vi "Camera.vi"(2 "Camera Queue":refnum<queue>, 3 "Wave Queue":refnum<queue>) -> (0 "error IO":errorcluster)   [LabVIEW 2016]
uses:
  controls/ModeEnum.ctl
  controls/Microscope Settings.ctl
  controls/ColourCalibration.ctl
  controls/CameraControlTypeDef.ctl
  controls/Stack_State.ctl
  controls/Stack Track.ctl
  <vilib>/vision/NI_Vision_Development_Module.lvlib
panel:
  out "Maximal Value":sgl
  in  "Display?":bool=TRUE
  out "Failed":bool
  out "Image":T1(plugin-control)
  out "FPS":dbl format="%#_3g"
  out "Image Path":path
  in  "Image Folder":path
  in  "Auto Contrast":bool
  out "Histogram":T2(graph)
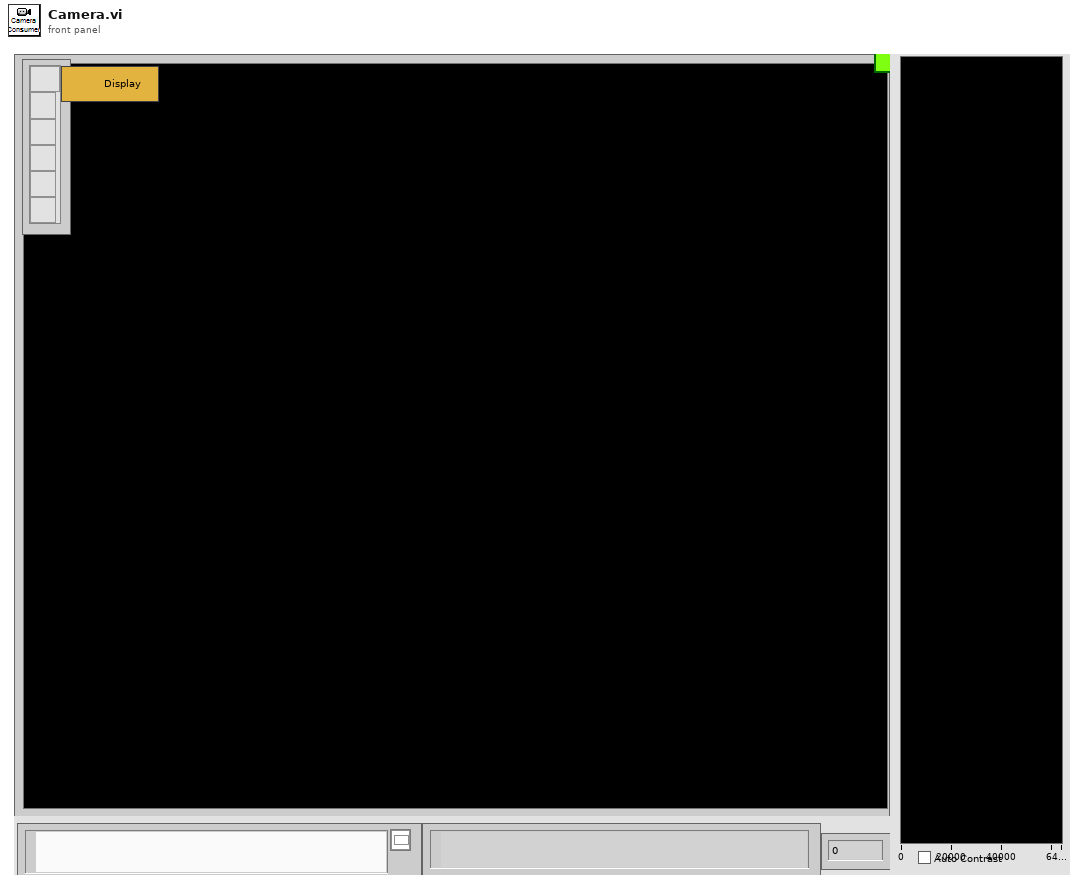
[diagram p1: front panel]
types:
  T1 = typedef "IMAQ Image.ctl" = refnum<image>
  T2 = cluster{"Starting Value":sgl, "Incremental Value":sgl, "Histogram":u32[]}
  T3 = typedef "Microscope Settings.ctl" = cluster{"Mode":enum16{"Brightfield", "X", "XY", "XYZ", "XYC", "XYCT", "XYZT", "XYZC", "Tweezers", "Virus"}, "Slit":cluster{"Scanning Mode":dbl, "Slit Width /%":dbl}, "Colour Channel":enum16{"1", "2", "3", "4", "5"}, "Colour":T4, "Exposure/ms":dbl, "Piezo Position /um":dbl, "ROI":cluster{"X":cluster{"Start /px":dbl, "Step /px":dbl, "Range /px":dbl}, "Y":cluster{"Start /px":dbl, "Step /px":dbl, "Range /px":dbl}, "Z ":cluster{"Start /um":dbl, "Step/um":dbl, "Range /um":dbl}, "T ":cluster{"Start /s":dbl, "Step /s":dbl, "Range /s":dbl}}, "Samples per millisecond":dbl, "Relax/ms":dbl, "Readout Direction":dbl, "Trigger Source":dbl, "Camera Delay /ms":dbl, "Under Scan /ms":dbl, "Slit Delay":dbl, "Waveforms":cluster{"Analogue Out":waveform(dbl)[], "Digital Out":digitalwaveform[]}}
  T4 = typedef "ColourCalibration.ctl" = cluster{"Colour":cluster{"Laser":enum16{"Brightfield", "445", "488", "561", "647"}, "Filter":u16}, "Calibration Coordinates":cluster{"Top Left":dbl[], "Top Right":dbl[], "Bottom Left":dbl[], "Bottom Right":dbl[]}, "Focus Offset /um":dbl}[]
  T5 = typedef "Image Type" = u32
  T6 = typedef "Stack_State.ctl" = cluster{"State":T7, "Image":u16[][], "Path":path}
  T7 = typedef "Stack Track.ctl" = enum16{"Idle", "STOP", "Display", "Save Image"}
  T8 = typedef "CameraControlTypeDef.ctl" = enum16{"Idle", "Init", "Close", "IntervalLineInt", "Ram Record", "HardDisk Record", "Disengage Update", "Update", "ROI", "Binning", "Scan Mode", "Trigger Mode", "Readout Mode", "Readout Direction", "Preview", "ROIWindow", "Trigger Source", "STOP"}
  T9 = cluster{"height":u32, "width":u32, "datatype":u32}
  T10 = typedef "ModeEnum.ctl" = enum16{"Idle", "Init", "generateWaves", "runWaves", "runWavesCont", "endWavesCont", "stop"}
  T11 = cluster{"Horizontal Offset":i32, "Vertical Offset":i32, "Horizontal Width":i32, "Vertical Width":i32}
  T12 = cluster{"Mode":u32, "Polarity":u32, "Times":u32, "Delay":dbl}
  T13 = cluster{"Start /px":dbl, "Step /px":dbl, "Range /px":dbl}
  T14 = cluster{"State":T7, "Data 16":u16[][], "Save to:":path}
  T15 = enum16{"Brightfield", "X", "XY", "XYZ", "XYC", "XYCT", "XYZT", "XYZC", "Tweezers", "Virus"}
  T16 = cluster{"histogram":u32[], "Minimal Value":sgl, "Maximal Value":sgl, "Starting Value":sgl, "Interval Width":sgl, "Mean Value":sgl, "Standard  Variation":sgl, "Area (pixels)":i32}
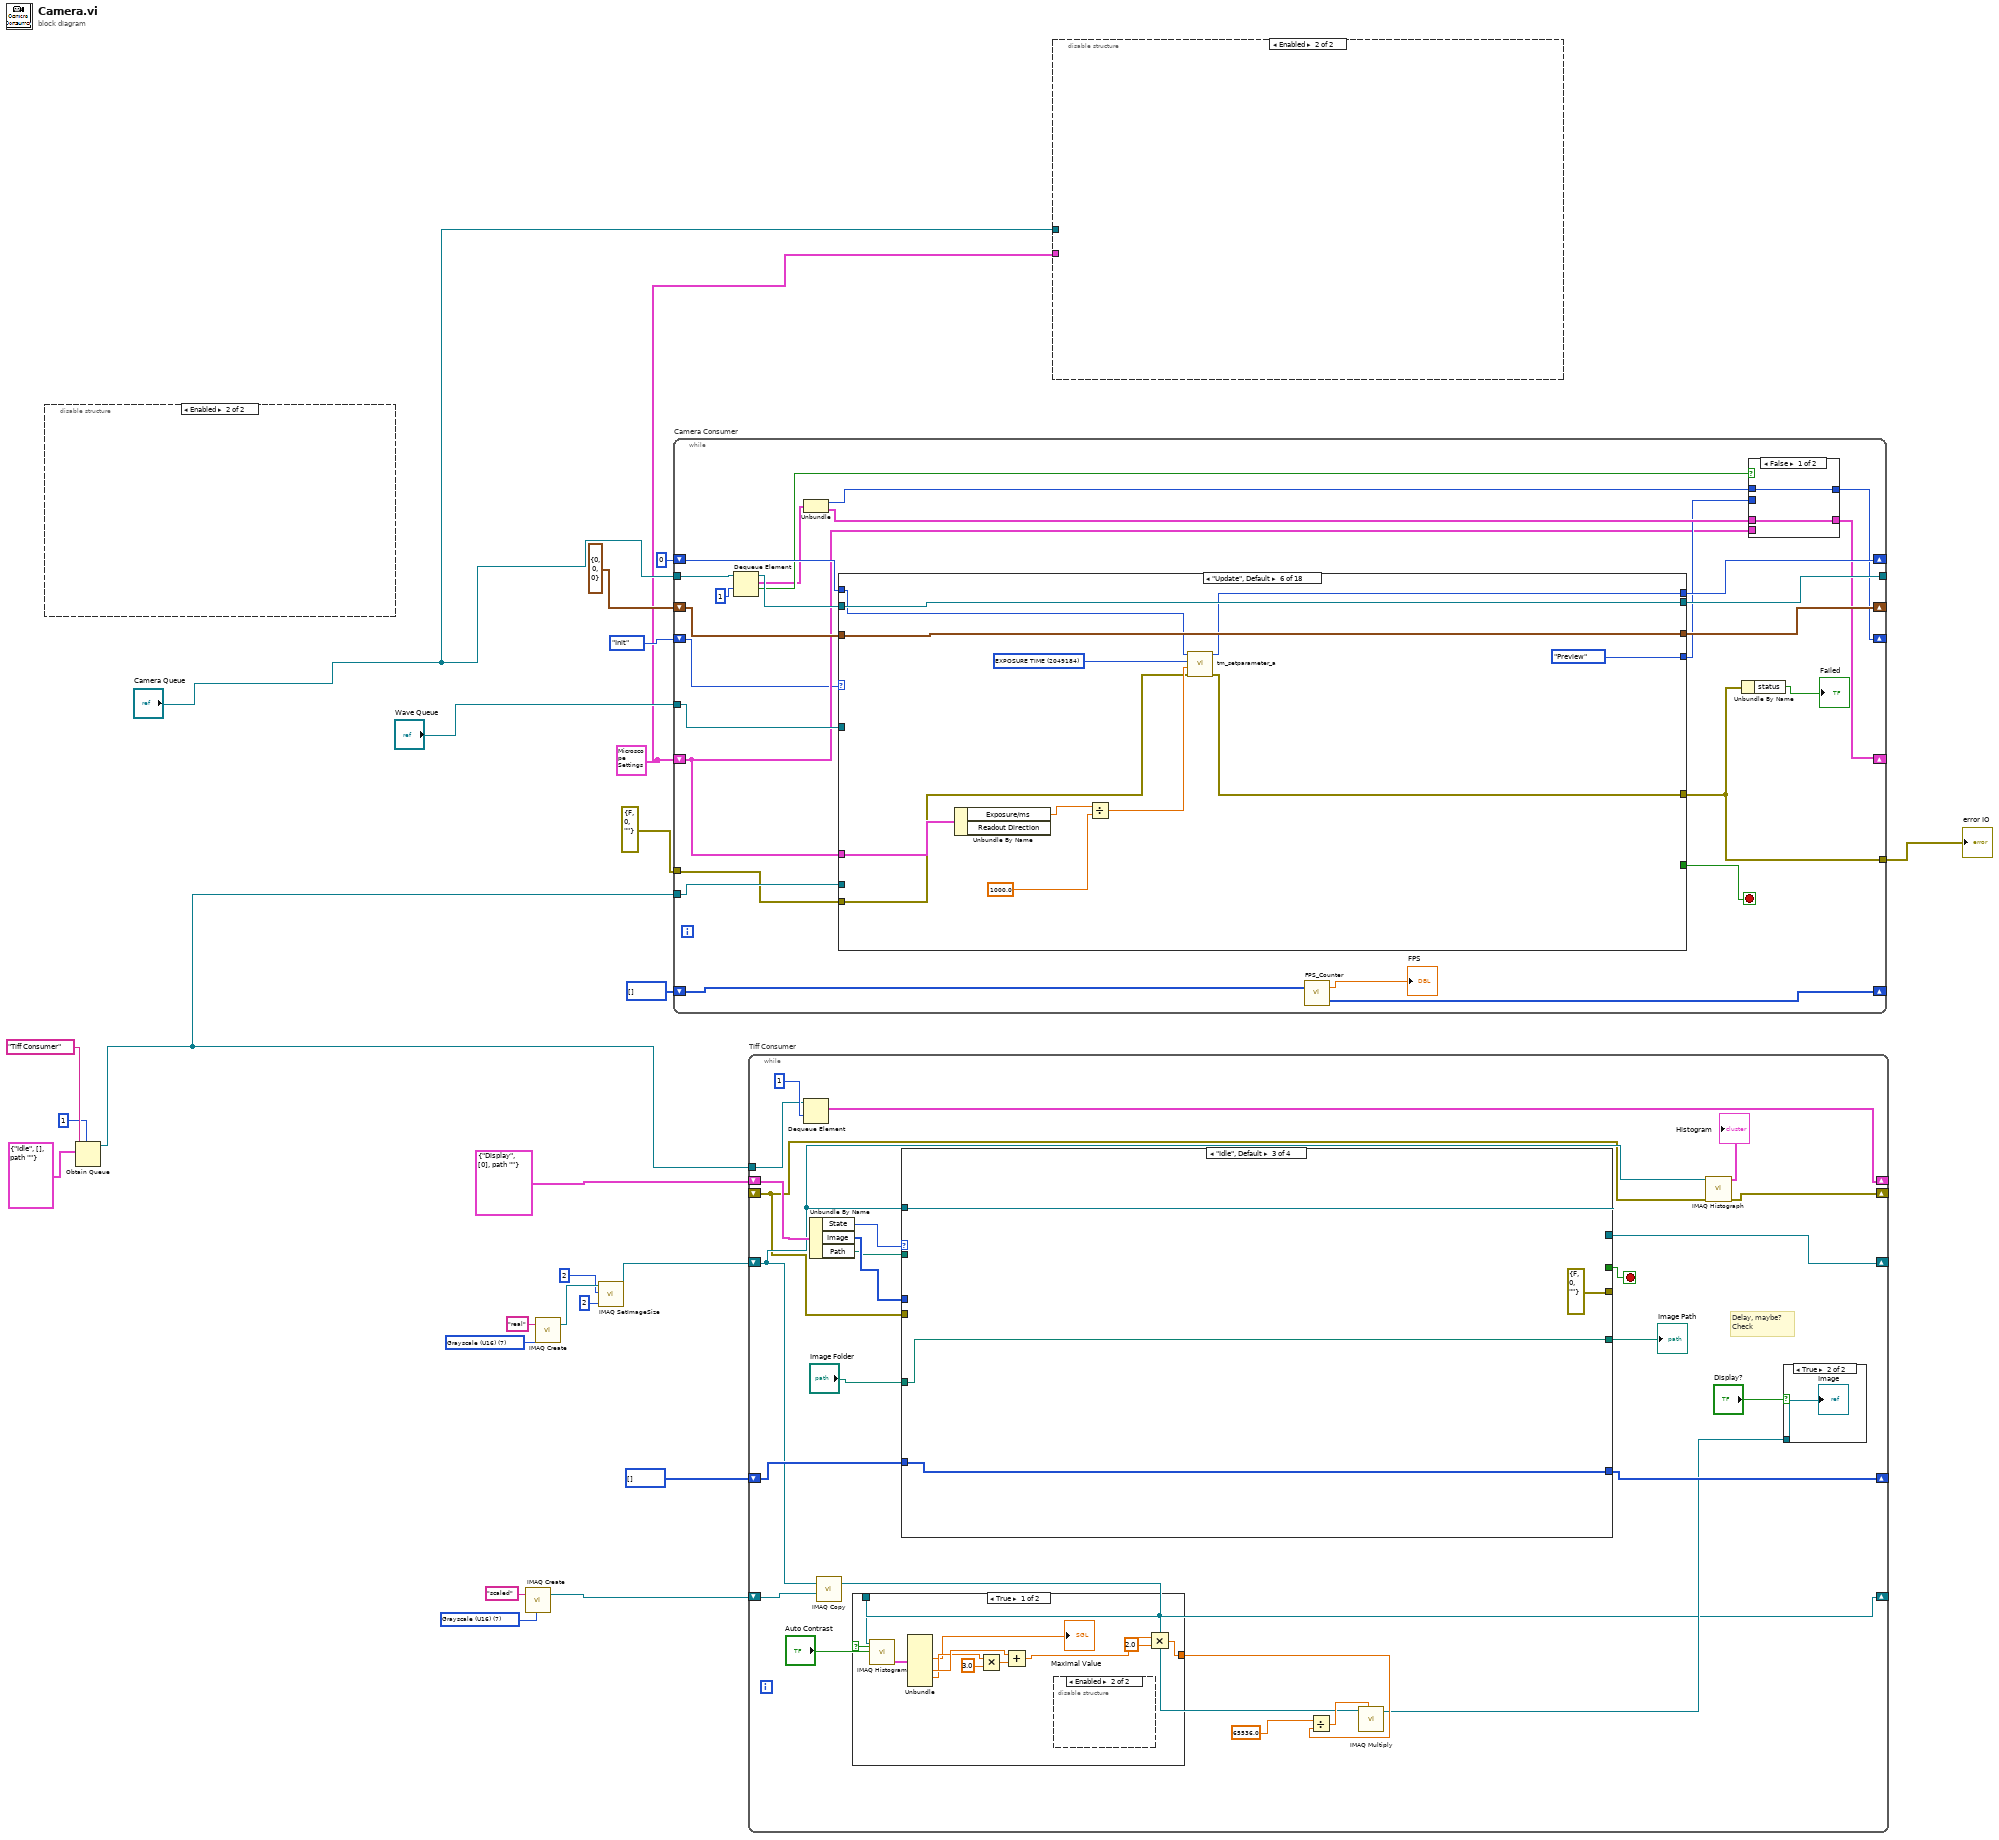
[diagram p0: block diagram]
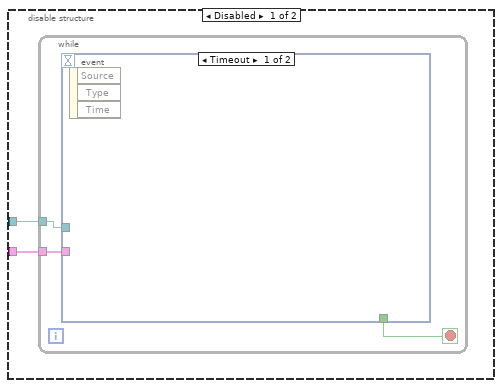
[diagram p2: hidden frame]
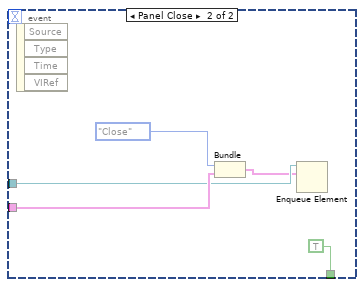
[diagram p3: hidden frame]
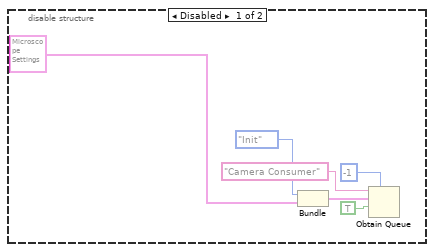
[diagram p4: hidden frame]
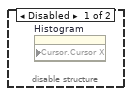
[diagram p5: hidden frame]
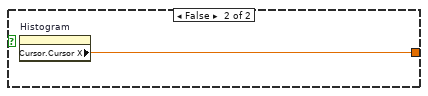
[diagram p6: hidden frame]
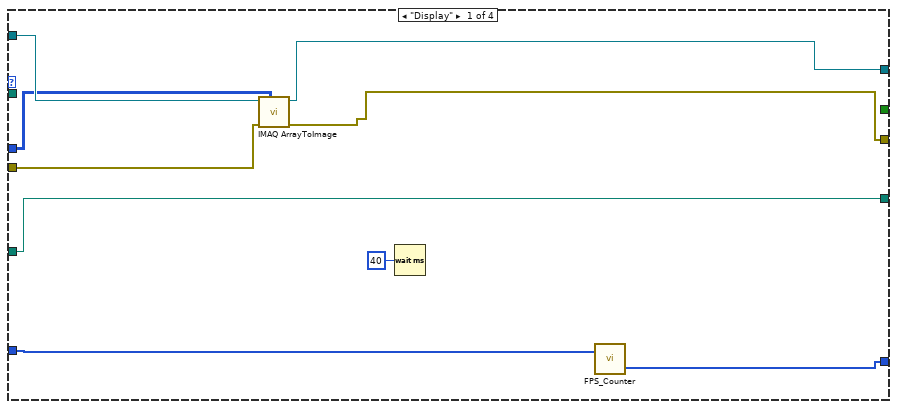
[diagram p8: hidden frame]
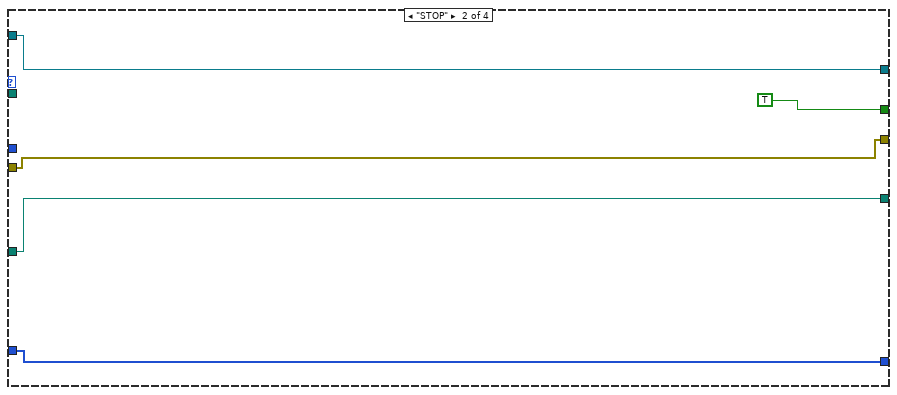
[diagram p9: hidden frame]
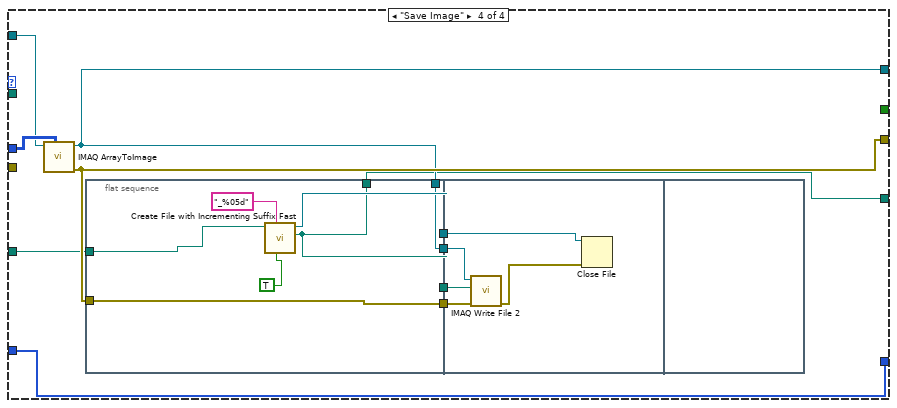
[diagram p10: hidden frame]
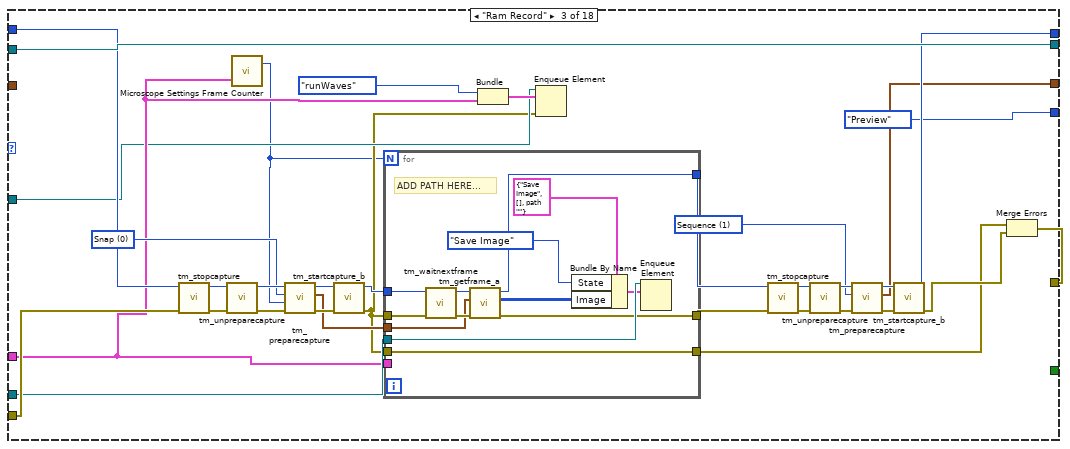
[diagram p13: hidden frame]
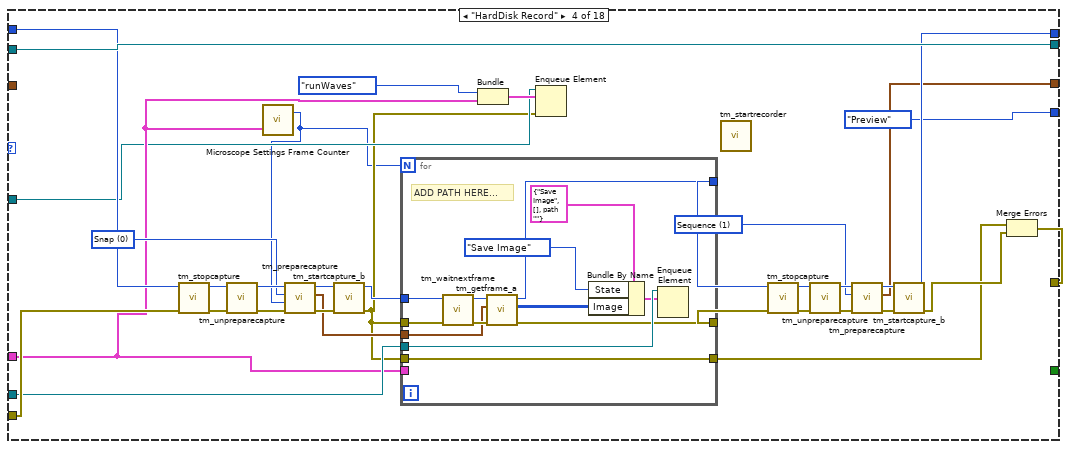
[diagram p14: hidden frame]
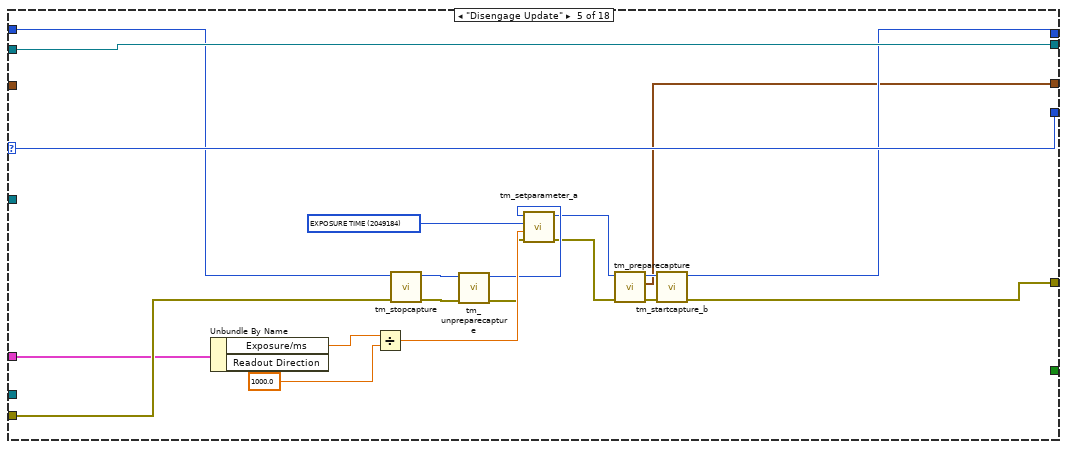
[diagram p15: hidden frame]
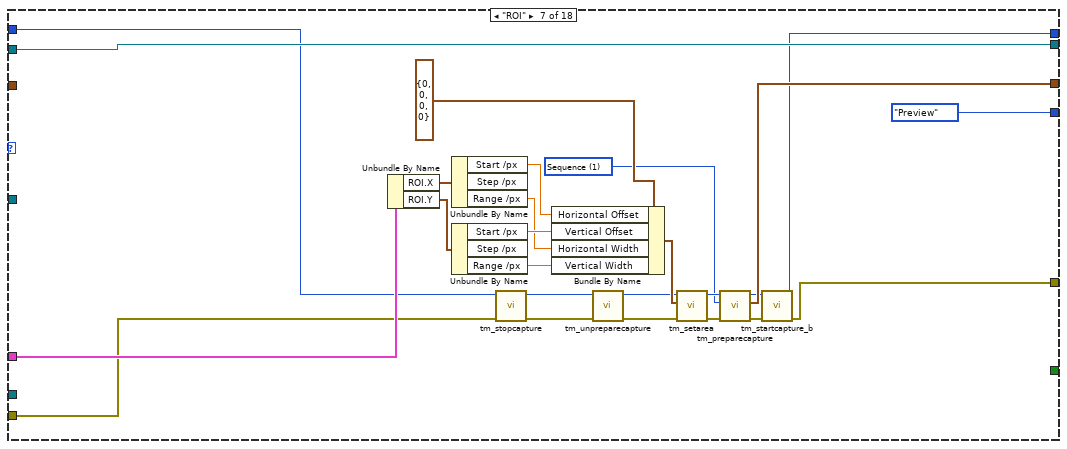
[diagram p16: hidden frame]
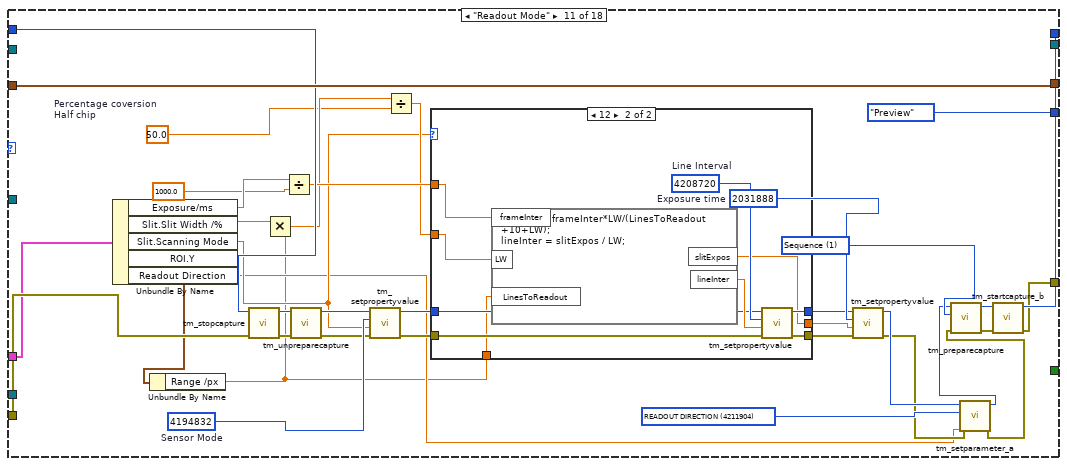
[diagram p20: hidden frame]
diagram:
  w1 = T3 {"Mode"=enum."X", "Slit"={"Scanning Mode"=12.0, "Slit Width /%"=5.0}, "Colour Channel"=enum."3", "Colour"=[], "Exposure/ms"=40.0, "Piezo Position /um"=10.0, "ROI"={"X"={"Start /px"=0.0, "Step /px"=1.0, "Range /px"=100.0}, "Y"={"Start /px"=0.0, "Step /px"=1.0, "Range /px"=100.0}, "Z "={"Start /um"=0.0, "Step/um"=1.0, "Range /um"=100.0}, "T "={"Start /s"=0.0, "Step /s"=1.0, "Range /s"=100.0}}, "Samples per millisecond"=100.0, "Relax/ms"=10000.0, "Readout Direction"=2.0, "Trigger Source"=2.0, "Camera Delay /ms"=11.0, "Under Scan /ms"=5.0, "Slit Delay"=100.0, "Waveforms"={"Analogue Out"=[{"t0"=timestamp(0 s since 1904-01-01), "dt"=1.0, "Y"=[]}, {"t0"=timestamp(0 s since 1904-01-01), "dt"=1.0, "Y"=[]}, {"t0"=timestamp(0 s since 1904-01-01), "dt"=1.0, "Y"=[]}], "Digital Out"=[{"t0"=timestamp(0 s since 1904-01-01), "dt"=0.0, "Y"={"transitions"=[], "data"=[]}}, {"t0"=timestamp(0 s since 1904-01-01), "dt"=0.0, "Y"={"transitions"=[], "data"=[]}}, {"t0"=timestamp(0 s since 1904-01-01), "dt"=0.0, "Y"={"transitions"=[], "data"=[]}}]}} ("Microscope Settings")
  w13 = T5 7 items=["Grayscale (U8)", "Grayscale (I16)", "Grayscale (SGL)", "Complex (CSG)", "RGB (U32)", "HSL (U32)", "RGB (U64)", "Grayscale (U16)"] ("Image Type")
  w24 = T5 7 items=["Grayscale (U8)", "Grayscale (I16)", "Grayscale (SGL)", "Complex (CSG)", "RGB (U32)", "HSL (U32)", "RGB (U64)", "Grayscale (U16)"] ("Image Type")
  n1 = disable-structure shown="Enabled" {
    frame Disabled {
      n2 = Bundle("Enum"=CameraControlTypeDef."Init", "Microscope Settings"=T3 {"Mode"=enum."X", "Slit"={"Scanning Mode"=12.0, "Slit Width /%"=5.0}, "Colour Channel"=enum."3", "Colour"=[{"Colour"={"Laser"=enum."561", "Filter"=4}, "Calibration Coordinates"={"Top Left"=[-4.418670520231216, -0.1592138728323702, 10.0], "Top Right"=[-9.501965317919073, -0.1592138728323702, 10.0], "Bottom Left"=[-4.4508670520231215, 0.0, 0.0], "Bottom Right"=[-9.53757225433526, 0.0, 0.0]}, "Focus Offset /um"=0.0}], "Exposure/ms"=40.0, "Piezo Position /um"=0.0, "ROI"={"X"={"Start /px"=0.0, "Step /px"=1.0, "Range /px"=2048.0}, "Y"={"Start /px"=0.0, "Step /px"=1.0, "Range /px"=2048.0}, "Z "={"Start /um"=0.0, "Step/um"=1.0, "Range /um"=100.0}, "T "={"Start /s"=0.0, "Step /s"=1.0, "Range /s"=100.0}}, "Samples per millisecond"=100.0, "Relax/ms"=10.0, "Readout Direction"=2.0, "Trigger Source"=2.0, "Camera Delay /ms"=11.0, "Under Scan /ms"=5.0, "Slit Delay"=100.0, "Waveforms"={"Analogue Out"=[{"t0"=timestamp(0 s since 1904-01-01), "dt"=1.0, "Y"=[]}, {"t0"=timestamp(0 s since 1904-01-01), "dt"=1.0, "Y"=[]}, {"t0"=timestamp(0 s since 1904-01-01), "dt"=1.0, "Y"=[]}], "Digital Out"=[{"t0"=timestamp(0 s since 1904-01-01), "dt"=0.0, "Y"={"transitions"=[], "data"=[]}}, {"t0"=timestamp(0 s since 1904-01-01), "dt"=0.0, "Y"={"transitions"=[], "data"=[]}}, {"t0"=timestamp(0 s since 1904-01-01), "dt"=0.0, "Y"={"transitions"=[], "data"=[]}}]}}) -> (w27:cluster{"Enum":T8, "Microscope Settings":T3})  [unwired: 1 in]
      n3 = Obtain Queue(max queue size (-1, unlimited)=-1, name (unnamed)="Camera Consumer", element data type=w27, create if not found? (T)=TRUE) -> ()  [unwired: 1 in, 3 out]
    }
    frame Enabled {
    }
  }
  n4 = Obtain Queue(max queue size (-1, unlimited)=1, name (unnamed)="Tiff Consumer", element data type=T6 {"State"=enum."Idle", "Image"=[], "Path"=path ""} ("input cluster")) -> (queue out=w14:refnum<queue>)  [unwired: 2 in, 2 out]
  n5 = call "IMAQ Create"("Image Name"="scaled", "Image Type"=w13) -> ("New Image"=w11:T1)  [unwired: 3 in, 1 out]
  n6 = call "IMAQ Create"("Image Name"="real", "Image Type"=w24) -> ("New Image"=w7:T1)  [unwired: 3 in, 1 out]
  n7 = call "IMAQ SetImageSize"("Y Resolution"=2, "X Resolution"=2, "Image"=w7) -> ("Image Out"=w6:T1)  [unwired: 2 in, 1 out]
  n8 = while "Camera Consumer" {
    tunnel: errorcluster {"status"=FALSE, "code"=0, "source"=""} ("error IO") -> [w42]
    tunnel: [w44] -> w17
    tunnel: "Camera Queue" -> [w50]
    tunnel: [w56] -> _
    shift-right: [w36] -> _
    shift-left: CameraControlTypeDef."Init" ("Enum") -> [w34]
    tunnel: w14 -> [w48]
    shift-right: [w54] -> _
    shift-left: u32 0 ("Handle out") -> [w55]
    tunnel: "Wave Queue" -> [w47]
    shift-right: [w53] -> _
    shift-left: T9 {"height"=0, "width"=0, "datatype"=0} ("Buffer Info") -> [w52]
    shift-right: [w37] -> _
    shift-left: w1 -> [w35]
    shift-right: [w32] -> _
    shift-left: u32[] [] ("Array out") -> [w33]
    stop <- w45 stop-if-true
    n9 = Dequeue Element(queue=w50, timeout in ms (-1)=1) -> (queue out=w49:refnum<queue>, element=w41:cluster{"Enum":T8, "Microscope Settings":T3}, timed out?=w46:bool)  [unwired: 1 in, 1 out]
    n10 = Unbundle(w41) -> ("Enum"=w40:T8, "Microscope Settings"=w39:T3)
    n11 = case shown="\"Update\", Default" w34 {
      selector: w34 -> [w60 w65 _ _ w179 _ _ w221 w226 w231 _ w287 _ w318 _ _ _ _]
      tunnel: w49 -> [w59 w66 w100 w147 w180 w192 w217 w222 w227 w232 _ w283 w299 w320 w331 w385 w405 w442]
      tunnel: [w59 w66 w100 w147 w180 w192 w217 w222 w227 w232 _ w283 w299 w320 w330 _ _ w442] -> w56
      tunnel: w42 -> [w61 w64 w99 w146 w171 w182 w195 w220 w225 w230 w265 w286 w292 w317 w321 w390 w410 w433]
      tunnel: [w61 w64 w77 w124 w170 w181 w198 w220 w225 w230 w242 w286 w291 w317 w334 w384 w404 w434] -> w44
      tunnel: [w60 w65 CameraControlTypeDef."Preview" ("Enum") CameraControlTypeDef."Preview" ("Enum") w179 CameraControlTypeDef."Preview" ("Enum") CameraControlTypeDef."Preview" ("Enum") w221 w226 w231 CameraControlTypeDef."Preview" ("Enum") w287 CameraControlTypeDef."Preview" ("Enum") w318 CameraControlTypeDef."Trigger Source" ("Enum") CameraControlTypeDef."Idle" ("Enum") CameraControlTypeDef."Idle" ("Enum") w424] -> w38
      tunnel: w55 -> [w58 w63 w83 w130 w174 w190 w197 w219 w224 w229 w267 w285 w298 w319 _ w381 w401 w436]
      tunnel: [w58 w63 w82 w129 w173 w189 w200 w219 w224 w229 w243 w285 w296 w319 w336 w381 w401 w435] -> w54
      tunnel: [w57 w62 w79 w126 w172 w191 w202 w218 w223 w228 w269 w284 w294 w316 w333 w382 w402 w437] -> w53
      tunnel: w52 -> [w57 w62 _ _ _ w191 _ w218 w223 w228 w269 w284 w294 w316 _ w382 w402 _]
      tunnel: w48 -> [_ _ w92 w139 _ _ _ _ _ _ _ _ w293 _ _ w375 w399 _]
      tunnel: w35 -> [_ _ w70 w117 w167 w188 w216 _ _ _ w264 _ _ _ w332 _ _ w426]
      tunnel: w47 -> [_ _ w69 w116 _ _ _ _ _ _ _ _ _ _ _ _ _ _]
      tunnel: [_ _ _ _ _ _ _ _ _ _ _ _ _ _ _ TRUE FALSE _] -> w45
      frame "Idle" {
      }
      frame "IntervalLineInt" {
      }
      frame "Ram Record" {
        w96 = 0 items=["Snap", "Sequence"] ("Capture mode")
        w80 = 1 items=["Snap", "Sequence"] ("Capture mode")
        n12 = call <userlib>:"tm_stopcapture.vi"("error in (no error)"=w99, "Handle in"=w83) -> ("error out"=w75:errorcluster, "Handle out"=w76:u32)  [unwired: 8 in]
        n13 = call <userlib>:"tm_unpreparecapture.vi"("error in (no error)"=w75, "Handle in"=w76) -> ("error out"=w98:errorcluster, "Handle out"=w97:u32)  [unwired: 8 in]
        n14 = call "Microscope Settings Frame Counter.vi"("Microscope Settings in"=w70) -> ("Camera Prepare"=w67:i32)  [unwired: 1 in, 1 out]
        n15 = call <userlib>:"tm_preparecapture.vi"("error in (no error)"=w98, "Frames"=w67, "Capture mode"=w96, "Handle in"=w97) -> ("error out"=w94:errorcluster, "Buffer Info"=w81:T9, "Handle out"=w95:u32)  [unwired: 4 in, 1 out]
        n16 = call <userlib>:"tm_startcapture_b.vi"("error in (no error)"=w94, "Handle in"=w95) -> ("error out"=w68:errorcluster, "Handle out"=w93:u32)  [unwired: 8 in]
        n17 = for {
          N: w67 -> [_]
          tunnel: w68 -> [w113]
          tunnel: w93 -> [w112]
          tunnel: w92 -> [w108]
          tunnel: [w106] -> w88
          tunnel: [w105] -> w87
          tunnel: w81 -> [w104]
          tunnel: w68 -> [w101]
          tunnel: w70 -> [_]
          tunnel: [w101] -> w74
          # "ADD PATH HERE..."
          n18 = call <userlib>:"tm_waitnextframe.vi"("error in (no error)"=w113, "Handle in"=w112) -> ("error out"=w111:errorcluster, "Handle out"=w110:u32)  [unwired: 6 in, 2 out]
          n19 = call <userlib>:"tm_getframe_a.vi"("error in (no error)"=w111, "Buffer Info"=w104, "Handle in"=w110) -> ("error out"=w106:errorcluster, "Data 16"=w103:u16[][], "Handle out"=w105:u32)  [unwired: 4 in, 2 out]
          n20 = Bundle By Name(cluster=T6 {"State"=enum."Save Image", "Image"=[], "Path"=path ""} ("element"), "State"=Stack_Track."Save Image", "Image"=w103) -> (w107:T6)
          n21 = Enqueue Element(queue=w108, element=w107) -> ()  [unwired: 2 in, 3 out]
        }
        n22 = Bundle("Mode"=ModeEnum."runWaves", "Microscope Settings"=w70) -> (w72:cluster{"Mode":T10, "Microscope Settings":T3})  [unwired: 1 in]
        n23 = Enqueue Element(queue=w69, element=w72, error in (no error)=w68) -> ()  [unwired: 1 in, 3 out]
        n24 = call <userlib>:"tm_stopcapture.vi"("error in (no error)"=w88, "Handle in"=w87) -> ("error out"=w89:errorcluster, "Handle out"=w86:u32)  [unwired: 8 in]
        n25 = call <userlib>:"tm_unpreparecapture.vi"("error in (no error)"=w89, "Handle in"=w86) -> ("error out"=w90:errorcluster, "Handle out"=w85:u32)  [unwired: 8 in]
        n26 = call <userlib>:"tm_preparecapture.vi"("error in (no error)"=w90, "Capture mode"=w80, "Handle in"=w85) -> ("error out"=w91:errorcluster, "Buffer Info"=w79:T9, "Handle out"=w84:u32)  [unwired: 5 in, 1 out]
        n27 = call <userlib>:"tm_startcapture_b.vi"("error in (no error)"=w91, "Handle in"=w84) -> ("error out"=w78:errorcluster, "Handle out"=w82:u32)  [unwired: 8 in]
        n28 = Merge Errors(w74, w78) -> (w77:errorcluster)
      }
      frame "HardDisk Record" {
        w143 = 0 items=["Snap", "Sequence"] ("Capture mode")
        w127 = 1 items=["Snap", "Sequence"] ("Capture mode")
        n29 = call <userlib>:"tm_stopcapture.vi"("error in (no error)"=w146, "Handle in"=w130) -> ("error out"=w122:errorcluster, "Handle out"=w123:u32)  [unwired: 8 in]
        n30 = call <userlib>:"tm_unpreparecapture.vi"("error in (no error)"=w122, "Handle in"=w123) -> ("error out"=w145:errorcluster, "Handle out"=w144:u32)  [unwired: 8 in]
        n31 = call "Microscope Settings Frame Counter.vi"("Microscope Settings in"=w117) -> ("Camera Prepare"=w114:i32)  [unwired: 1 in, 1 out]
        n32 = call <userlib>:"tm_preparecapture.vi"("error in (no error)"=w145, "Frames"=w114, "Capture mode"=w143, "Handle in"=w144) -> ("error out"=w141:errorcluster, "Buffer Info"=w128:T9, "Handle out"=w142:u32)  [unwired: 4 in, 1 out]
        n33 = call <userlib>:"tm_startcapture_b.vi"("error in (no error)"=w141, "Handle in"=w142) -> ("error out"=w115:errorcluster, "Handle out"=w140:u32)  [unwired: 8 in]
        n34 = for {
          N: w114 -> [_]
          tunnel: w115 -> [w160]
          tunnel: w140 -> [w159]
          tunnel: w139 -> [w155]
          tunnel: [w153] -> w135
          tunnel: [w152] -> w134
          tunnel: w128 -> [w151]
          tunnel: w115 -> [w148]
          tunnel: w117 -> [_]
          tunnel: [w148] -> w121
          # "ADD PATH HERE..."
          n35 = call <userlib>:"tm_waitnextframe.vi"("error in (no error)"=w160, "Handle in"=w159) -> ("error out"=w158:errorcluster, "Handle out"=w157:u32)  [unwired: 6 in, 2 out]
          n36 = call <userlib>:"tm_getframe_a.vi"("error in (no error)"=w158, "Buffer Info"=w151, "Handle in"=w157) -> ("error out"=w153:errorcluster, "Data 16"=w150:u16[][], "Handle out"=w152:u32)  [unwired: 4 in, 2 out]
          n37 = Bundle By Name(cluster=T6 {"State"=enum."Save Image", "Image"=[], "Path"=path ""} ("element"), "State"=Stack_Track."Save Image", "Image"=w150) -> (w154:T6)
          n38 = Enqueue Element(queue=w155, element=w154) -> ()  [unwired: 2 in, 3 out]
        }
        n39 = Bundle("Mode"=ModeEnum."runWaves", "Microscope Settings"=w117) -> (w119:cluster{"Mode":T10, "Microscope Settings":T3})  [unwired: 1 in]
        n40 = Enqueue Element(queue=w116, element=w119, error in (no error)=w115) -> ()  [unwired: 1 in, 3 out]
        n41 = call <userlib>:"tm_startrecorder.vi"() -> ()  [unwired: 10 in, 2 out]
        n42 = call <userlib>:"tm_stopcapture.vi"("error in (no error)"=w135, "Handle in"=w134) -> ("error out"=w136:errorcluster, "Handle out"=w133:u32)  [unwired: 8 in]
        n43 = call <userlib>:"tm_unpreparecapture.vi"("error in (no error)"=w136, "Handle in"=w133) -> ("error out"=w137:errorcluster, "Handle out"=w132:u32)  [unwired: 8 in]
        n44 = call <userlib>:"tm_preparecapture.vi"("error in (no error)"=w137, "Capture mode"=w127, "Handle in"=w132) -> ("error out"=w138:errorcluster, "Buffer Info"=w126:T9, "Handle out"=w131:u32)  [unwired: 5 in, 1 out]
        n45 = call <userlib>:"tm_startcapture_b.vi"("error in (no error)"=w138, "Handle in"=w131) -> ("error out"=w125:errorcluster, "Handle out"=w129:u32)  [unwired: 8 in]
        n46 = Merge Errors(w121, w125) -> (w124:errorcluster)
      }
      frame "Disengage Update" {
        w169 = u32 2049184 items=["SENSOR MODE"=4212128, "CCD MODE"=4212384, "READOUT MODE"=4211872, "ACTIVE VIEW INDEX"=4343136, "BITS PER CHANNEL"=4342976, "IMAGE PIXEL TYPE"=4343296, "BINNING"=4215968, "EXPOSURE TIME"=2049184, "CONTRAST GAIN"=3163312, "CONTRAST OFFSET"=3163328, "LIGHT MODE"=2114720, "SENSITIVITY"=2114992, "PHOTON IMAGING MODE"=2115200, "HIGH DYNAMIC RANGE MODE"=3163360, "WHITE BALANCE"=3163568, "TEMPERATURE"=2115232, "TEMPERATURE TARGET"=2115264, "SENSOR COOLER FAN"=2115296, "LINEBUNDLE HEIGHT"=4212192, "MECHANICAL SHUTTER"=2115488, "BACK FOCUS POSITION"=8422304, "TRIGGER CONNECTOR"=1066432, "TRIGGER SOURCE"=1066144, "OUTPUT TRIGGER SOURCE"=1852576, "TRIGGER GLOBAL EXPOSURE"=2049680, "FIRST TRIGGER BEHAVIOR"=2049696, "CHANNEL SYNC"=1852352, "READOUT DIRECTION"=4211904, "PRE HSYNC COUNT"=1852704, "INTERNAL LINE SPEED"=4226000, "INTERNAL LINE INTERVAL"=4226016] ("Parameter")
        n47 = Unbundle By Name(w167) -> ("Exposure/ms"=w166:dbl)  [unwired: 1 out]
        n48 = Divide(x=w166, y=1000.0) -> (x/y=w165:dbl)
        n49 = call <userlib>:"tm_stopcapture.vi"("error in (no error)"=w171, "Handle in"=w174) -> ("error out"=w177:errorcluster, "Handle out"=w176:u32)  [unwired: 8 in]
        n50 = call <userlib>:"tm_unpreparecapture.vi"("error in (no error)"=w177, "Handle in"=w176) -> ("error out"=w161:errorcluster, "Handle out"=w164:u32)  [unwired: 8 in]
        n51 = call <userlib>:"tm_setparameter_a.vi"("error in (no error)"=w161, "Value in"=w165, "Parameter"=w169, "Handle in"=w164) -> ("error out"=w162:errorcluster, "Handle out"=w163:u32)  [unwired: 6 in]
        n52 = call <userlib>:"tm_preparecapture.vi"("error in (no error)"=w162, "Handle in"=w163) -> ("error out"=w178:errorcluster, "Buffer Info"=w172:T9, "Handle out"=w175:u32)  [unwired: 6 in, 1 out]
        n53 = call <userlib>:"tm_startcapture_b.vi"("error in (no error)"=w178, "Handle in"=w175) -> ("error out"=w170:errorcluster, "Handle out"=w173:u32)  [unwired: 8 in]
      }
      frame "Update", Default {
        w185 = u32 2049184 items=["SENSOR MODE"=4212128, "CCD MODE"=4212384, "READOUT MODE"=4211872, "ACTIVE VIEW INDEX"=4343136, "BITS PER CHANNEL"=4342976, "IMAGE PIXEL TYPE"=4343296, "BINNING"=4215968, "EXPOSURE TIME"=2049184, "CONTRAST GAIN"=3163312, "CONTRAST OFFSET"=3163328, "LIGHT MODE"=2114720, "SENSITIVITY"=2114992, "PHOTON IMAGING MODE"=2115200, "HIGH DYNAMIC RANGE MODE"=3163360, "WHITE BALANCE"=3163568, "TEMPERATURE"=2115232, "TEMPERATURE TARGET"=2115264, "SENSOR COOLER FAN"=2115296, "LINEBUNDLE HEIGHT"=4212192, "MECHANICAL SHUTTER"=2115488, "BACK FOCUS POSITION"=8422304, "TRIGGER CONNECTOR"=1066432, "TRIGGER SOURCE"=1066144, "OUTPUT TRIGGER SOURCE"=1852576, "TRIGGER GLOBAL EXPOSURE"=2049680, "FIRST TRIGGER BEHAVIOR"=2049696, "CHANNEL SYNC"=1852352, "READOUT DIRECTION"=4211904, "PRE HSYNC COUNT"=1852704, "INTERNAL LINE SPEED"=4226000, "INTERNAL LINE INTERVAL"=4226016] ("Parameter")
        n54 = Unbundle By Name(w188) -> ("Exposure/ms"=w187:dbl)  [unwired: 1 out]
        n55 = Divide(x=w187, y=1000.0) -> (x/y=w184:dbl)
        n56 = call <userlib>:"tm_setparameter_a.vi"("error in (no error)"=w182, "Value in"=w184, "Parameter"=w185, "Handle in"=w190) -> ("error out"=w181:errorcluster, "Handle out"=w189:u32)  [unwired: 6 in]
      }
      frame "ROI" {
        w205 = 1 items=["Snap", "Sequence"] ("Capture mode")
        n57 = Unbundle By Name(w216) -> ("ROI.X"=w215:T13, "ROI.Y"=w214:T13)
        n58 = Unbundle By Name(w215) -> ("Start /px"=w212:dbl, "Range /px"=w210:dbl)  [unwired: 1 out]
        n59 = Unbundle By Name(w214) -> ("Start /px"=w211:dbl, "Range /px"=w209:dbl)  [unwired: 1 out]
        n60 = call <userlib>:"tm_stopcapture.vi"("error in (no error)"=w195, "Handle in"=w197) -> ("error out"=w194:errorcluster, "Handle out"=w196:u32)  [unwired: 8 in]
        n61 = Bundle By Name(cluster=T11 {"Horizontal Offset"=0, "Vertical Offset"=0, "Horizontal Width"=0, "Vertical Width"=0} ("Sub Region"), "Horizontal Offset"=w212, "Vertical Offset"=w211, "Horizontal Width"=w210, "Vertical Width"=w209) -> (w208:T11)
        n62 = call <userlib>:"tm_unpreparecapture.vi"("error in (no error)"=w194, "Handle in"=w196) -> ("error out"=w203:errorcluster, "Handle out"=w207:u32)  [unwired: 8 in]
        n63 = call <userlib>:"tm_setarea.vi"("error in (no error)"=w203, "Sub Region"=w208, "Handle in"=w207) -> ("error out"=w204:errorcluster, "Handle out"=w206:u32)  [unwired: 7 in]
        n64 = call <userlib>:"tm_preparecapture.vi"("error in (no error)"=w204, "Capture mode"=w205, "Handle in"=w206) -> ("error out"=w199:errorcluster, "Buffer Info"=w202:T9, "Handle out"=w201:u32)  [unwired: 5 in, 1 out]
        n65 = call <userlib>:"tm_startcapture_b.vi"("error in (no error)"=w199, "Handle in"=w201) -> ("error out"=w198:errorcluster, "Handle out"=w200:u32)  [unwired: 8 in]
      }
      frame "Binning" {
      }
      frame "Scan Mode" {
      }
      frame "Trigger Mode" {
      }
      frame "Readout Mode" {
        w239 = u32 4211904 items=["SENSOR MODE"=4212128, "CCD MODE"=4212384, "READOUT MODE"=4211872, "ACTIVE VIEW INDEX"=4343136, "BITS PER CHANNEL"=4342976, "IMAGE PIXEL TYPE"=4343296, "BINNING"=4215968, "EXPOSURE TIME"=2049184, "CONTRAST GAIN"=3163312, "CONTRAST OFFSET"=3163328, "LIGHT MODE"=2114720, "SENSITIVITY"=2114992, "PHOTON IMAGING MODE"=2115200, "HIGH DYNAMIC RANGE MODE"=3163360, "WHITE BALANCE"=3163568, "TEMPERATURE"=2115232, "TEMPERATURE TARGET"=2115264, "SENSOR COOLER FAN"=2115296, "LINEBUNDLE HEIGHT"=4212192, "MECHANICAL SHUTTER"=2115488, "BACK FOCUS POSITION"=8422304, "TRIGGER CONNECTOR"=1066432, "TRIGGER SOURCE"=1066144, "OUTPUT TRIGGER SOURCE"=1852576, "TRIGGER GLOBAL EXPOSURE"=2049680, "FIRST TRIGGER BEHAVIOR"=2049696, "CHANNEL SYNC"=1852352, "READOUT DIRECTION"=4211904, "PRE HSYNC COUNT"=1852704, "INTERNAL LINE SPEED"=4191408, "INTERNAL LINE INTERVAL"=4191424] ("Parameter")
        w246 = 1 items=["Snap", "Sequence"] ("Capture mode")
        w252 = u32 4194832  # Sensor Mode
        w258 = 50.0  # Percentage coversion Half chip
        w255 = u32 2031888  # Exposure time
        n66 = Unbundle By Name(w264) -> ("Exposure/ms"=w263:dbl, "Slit.Slit Width /%"=w260:dbl, "Slit.Scanning Mode"=w250:dbl, "ROI.Y"=w240:T13, "Readout Direction"=w234:dbl)
        n67 = Unbundle By Name(w240) -> ("Range /px"=w233:dbl)
        n68 = call <userlib>:"tm_stopcapture.vi"("error in (no error)"=w265, "Handle in"=w267) -> ("error out"=w268:errorcluster, "Handle out"=w266:u32)  [unwired: 8 in]
        n69 = Multiply(x=w260, y=w233) -> (x*y=w259:dbl)
        n70 = Divide(x=w263, y=1000.0) -> (x/y=w261:dbl)
        n71 = call <userlib>:"tm_unpreparecapture.vi"("error in (no error)"=w268, "Handle in"=w266) -> ("error out"=w247:errorcluster, "Handle out"=w251:u32)  [unwired: 8 in]
        n72 = call "tm_setpropertyvalue.vi"("error in (no error)"=w247, "Value in"=w250, "Property ID"=w252, "Handle in"=w251) -> ("error out"=w248:errorcluster, "Handle out"=w249:u32)  [unwired: 6 in]
        n73 = Divide(x=w259, y=w258) -> (x/y=w257:dbl)
        n74 = case shown="12" w250 {
          tunnel: [w272 w274] -> w256
          tunnel: w261 -> [w272 w282]
          tunnel: w257 -> [_ w281]
          tunnel: w249 -> [w271 w276]
          tunnel: [w271 w278] -> w254
          tunnel: [w270 w277] -> w253
          tunnel: w248 -> [w270 w275]
          tunnel: w233 -> [_ w273]
          frame 1, Default {
          }
          frame 12 {
            w280 = u32 4208720  # Line Interval
            n75 = formula code="slitExpos=frameInter*LW/(LinesToReadout\n+10+LW);\nlineInter = slitExpos / LW;"("frameInter"=w282, "LW"=w281, "LinesToReadout"=w273) -> ("slitExpos"=w274:dbl, "lineInter"=w279:dbl)
            n76 = call "tm_setpropertyvalue.vi"("error in (no error)"=w275, "Value in"=w279, "Property ID"=w280, "Handle in"=w276) -> ("error out"=w277:errorcluster, "Handle out"=w278:u32)  [unwired: 6 in]
          }
        }
        n77 = call "tm_setpropertyvalue.vi"("error in (no error)"=w253, "Value in"=w256, "Property ID"=w255, "Handle in"=w254) -> ("error out"=w236:errorcluster, "Handle out"=w238:u32)  [unwired: 6 in]
        n78 = call <userlib>:"tm_setparameter_a.vi"("error in (no error)"=w236, "Value in"=w234, "Parameter"=w239, "Handle in"=w238) -> ("error out"=w235:errorcluster, "Handle out"=w237:u32)  [unwired: 6 in]
        n79 = call <userlib>:"tm_preparecapture.vi"("error in (no error)"=w235, "Capture mode"=w246, "Handle in"=w237) -> ("error out"=w245:errorcluster, "Handle out"=w244:u32)  [unwired: 5 in, 2 out]
        n80 = call <userlib>:"tm_startcapture_b.vi"("error in (no error)"=w245, "Handle in"=w244) -> ("error out"=w242:errorcluster, "Handle out"=w243:u32)  [unwired: 8 in]
      }
      frame "Readout Direction" {
      }
      frame "Preview" {
        n81 = call <userlib>:"tm_waitnextframe.vi"("error in (no error)"=w292, "Timeout"=500, "Handle in"=w298) -> ("error out"=w290:errorcluster, "Frame Index"=w289:i32, "Handle out"=w297:u32)  [unwired: 5 in, 1 out]
        n82 = case shown="No Error" w290 {
          selector: w290 -> [w303 w315]
          tunnel: w297 -> [w307 w314]
          tunnel: [w306 w314] -> w296
          tunnel: w294 -> [w305 _]
          tunnel: w293 -> [w304 _]
          tunnel: [w302 w315] -> w291
          tunnel: w289 -> [w301 _]
          frame No Error {
            n83 = call <userlib>:"tm_getframe_a.vi"("error in (no error)"=w303, "Frame Index"=w301, "Buffer Info"=w305, "Handle in"=w307) -> ("error out"=w302:errorcluster, "Data 16"=w300:u16[][], "Handle out"=w306:u32)  [unwired: 3 in, 2 out]
            n84 = disable-structure shown="Enabled" {
              disable-tunnel: w304 -> [w309 _]
              disable-tunnel: w300 -> [w310 _]
              frame Enabled {
                n85 = Flush Queue(queue=w309) -> (queue out=w308:refnum<queue>)  [unwired: 1 in, 2 out]
                n86 = Bundle("State"=Stack_Track."Display", "Data 16"=w310, "Save to:"=path "") -> (w311:T14)  [unwired: 1 in]
                n87 = Lossy Enqueue Element(queue=w308, element=w311) -> ()  [unwired: 1 in, 4 out]
              }
              frame Disabled {
              }
            }
          }
          frame Error {
          }
        }
      }
      frame "ROIWindow" {
      }
      frame "Init" {
        w339 = 1 items=["Snap", "Sequence"] ("Capture mode")
        n88 = call <userlib>:"tm_deinitialize.vi"("error in (no error)"=w321) -> ("error out"=w322:errorcluster)  [unwired: 10 in]
        n89 = call <userlib>:"tm_initialize.vi"("error in (no error)"=w322) -> ("error out"=w342:errorcluster)  [unwired: 7 in, 3 out]
        n90 = call <userlib>:"tm_opencamera.vi"("Force Open"=TRUE, "error in (no error)"=w342, "Camera Index"=u32 0) -> ("error out"=w341:errorcluster, "Handle out"=w340:u32)  [unwired: 6 in, 1 out]
        n91 = disable-structure shown="Enabled" {
          disable-tunnel: w341 -> [w346 w373]
          disable-tunnel: w340 -> [w347 w374]
          disable-tunnel: [w349 w374] -> w327
          disable-tunnel: [w348 w373] -> w324
          disable-tunnel: w332 -> [w354 _]
          frame Enabled {
            w353 = u32 4211872 items=["SENSOR MODE"=4212128, "CCD MODE"=4212384, "READOUT MODE"=4211872, "ACTIVE VIEW INDEX"=4343136, "BITS PER CHANNEL"=4342976, "IMAGE PIXEL TYPE"=4343296, "BINNING"=4215968, "EXPOSURE TIME"=2049184, "CONTRAST GAIN"=3163312, "CONTRAST OFFSET"=3163328, "LIGHT MODE"=2114720, "SENSITIVITY"=2114992, "PHOTON IMAGING MODE"=2115200, "HIGH DYNAMIC RANGE MODE"=3163360, "WHITE BALANCE"=3163568, "TEMPERATURE"=2115232, "TEMPERATURE TARGET"=2115264, "SENSOR COOLER FAN"=2115296, "LINEBUNDLE HEIGHT"=4212192, "MECHANICAL SHUTTER"=2115488, "BACK FOCUS POSITION"=8422304, "TRIGGER CONNECTOR"=1066432, "TRIGGER SOURCE"=1066144, "OUTPUT TRIGGER SOURCE"=1852576, "TRIGGER GLOBAL EXPOSURE"=2049680, "FIRST TRIGGER BEHAVIOR"=2049696, "CHANNEL SYNC"=1852352, "READOUT DIRECTION"=4211904, "PRE HSYNC COUNT"=1852704, "INTERNAL LINE SPEED"=4226000, "INTERNAL LINE INTERVAL"=4226016] ("Parameter")
            w360 = u32 2115296 items=["SENSOR MODE"=4212128, "CCD MODE"=4212384, "READOUT MODE"=4211872, "ACTIVE VIEW INDEX"=4343136, "BITS PER CHANNEL"=4342976, "IMAGE PIXEL TYPE"=4343296, "BINNING"=4215968, "EXPOSURE TIME"=2049184, "CONTRAST GAIN"=3163312, "CONTRAST OFFSET"=3163328, "LIGHT MODE"=2114720, "SENSITIVITY"=2114992, "PHOTON IMAGING MODE"=2115200, "HIGH DYNAMIC RANGE MODE"=3163360, "WHITE BALANCE"=3163568, "TEMPERATURE"=2115232, "TEMPERATURE TARGET"=2115264, "SENSOR COOLER FAN"=2115296, "LINEBUNDLE HEIGHT"=4212192, "MECHANICAL SHUTTER"=2115488, "BACK FOCUS POSITION"=8422304, "TRIGGER CONNECTOR"=1066432, "TRIGGER SOURCE"=1066144, "OUTPUT TRIGGER SOURCE"=1852576, "TRIGGER GLOBAL EXPOSURE"=2049680, "FIRST TRIGGER BEHAVIOR"=2049696, "CHANNEL SYNC"=1852352, "READOUT DIRECTION"=4211904, "PRE HSYNC COUNT"=1852704, "INTERNAL LINE SPEED"=4226000, "INTERNAL LINE INTERVAL"=4226016] ("Parameter")
            w365 = u32 2031888  # Exposure
            n92 = Unbundle By Name(w354) -> ("Exposure/ms"=w355:dbl, "Readout Direction"=w345:dbl)
            n93 = call "tm_setpropertyvalue.vi"("error in (no error)"=w346, "Value in"=sgl 1.0, "Property ID"=u32 4194832, "Handle in"=w347) -> ("error out"=w358:errorcluster, "Handle out"=w368:u32)  [unwired: 6 in]
            n94 = call "tm_setpropertyvalue.vi"("error in (no error)"=w358, "Value in"=sgl 1.0, "Property ID"=u32 1049104, "Handle in"=w368) -> ("error out"=w357:errorcluster, "Handle out"=w366:u32)  [unwired: 6 in]
            n95 = call <userlib>:"tm_setinputtrigger.vi"("error in (no error)"=w357, "Parameters"=T12 {"Mode"=1, "Polarity"=2, "Times"=1, "Delay"=0.0}, "Handle in"=w366) -> ("error out"=w356:errorcluster, "Handle out"=w364:u32)  [unwired: 7 in]
            n96 = Divide(x=w355, y=sgl 1000.0) -> (x/y=w362:dbl)
            n97 = call "tm_setpropertyvalue.vi"("error in (no error)"=w356, "Value in"=w362, "Property ID"=w365, "Handle in"=w364) -> ("error out"=w352:errorcluster, "Handle out"=w361:u32)  [unwired: 6 in]
            n98 = call <userlib>:"tm_setparameter_a.vi"("error in (no error)"=w352, "Value in"=2.0, "Parameter"=w360, "Handle in"=w361) -> ("error out"=w351:errorcluster, "Handle out"=w350:u32)  [unwired: 6 in]
            n99 = call <userlib>:"tm_setparameter_a.vi"("error in (no error)"=w351, "Value in"=w345, "Parameter"=w353, "Handle in"=w350) -> ("error out"=w348:errorcluster, "Handle out"=w349:u32)  [unwired: 6 in]
          }
          frame Disabled {
          }
        }
        n100 = Bundle("Enum"=CameraControlTypeDef."Trigger Source", "Microscope Settings"=w332) -> (w329:cluster{"Enum":T8, "Microscope Settings":T3})  [unwired: 1 in]
        n101 = Enqueue Element(queue=w331, element=w329) -> (queue out=w330:refnum<queue>)  [unwired: 2 in, 2 out]
        n102 = call "tm_setcooling.vi"("error in (no error)"=w324, "Mode"=TRUE, "Handle in"=w327) -> ("error out"=w323:errorcluster, "Handle out"=w325:u32)  [unwired: 7 in]
        n103 = call <userlib>:"tm_preparecapture.vi"("error in (no error)"=w323, "Capture mode"=w339, "Handle in"=w325) -> ("error out"=w338:errorcluster, "Buffer Info"=w333:T9, "Handle out"=w337:u32)  [unwired: 5 in, 1 out]
        n104 = call <userlib>:"tm_startcapture_b.vi"("error in (no error)"=w338, "Handle in"=w337) -> ("error out"=w334:errorcluster, "Handle out"=w336:u32)  [unwired: 8 in]
      }
      frame "Close" {
        n105 = Bundle("State"=Stack_Track."STOP", "Data 16"=u16[][] [], "Save to:"=path "C:/_DATA/test.tiff") -> (w377:T14)  [unwired: 1 in]
        n106 = Enqueue Element(queue=w375, element=w377) -> ()  [unwired: 2 in, 3 out]
        n107 = call <userlib>:"tm_stopcapture.vi"("error in (no error)"=w390) -> ("error out"=w389:errorcluster, "Handle out"=w392:u32)  [unwired: 9 in]
        n108 = call <userlib>:"tm_unpreparecapture.vi"("error in (no error)"=w389, "Handle in"=w392) -> ("error out"=w388:errorcluster, "Handle out"=w391:u32)  [unwired: 8 in]
        n109 = call <userlib>:"tm_closecamera.vi"("error in (no error)"=w388, "Handle in"=w391) -> ("error out"=w387:errorcluster)  [unwired: 9 in]
        n110 = call <userlib>:"tm_deinitialize.vi"("error in (no error)"=w387) -> ("error out"=w386:errorcluster)  [unwired: 10 in]
        n111 = disable-structure shown="Enabled" {
          disable-tunnel: w386 -> [w397 w398]
          disable-tunnel: w385 -> [w394 _]
          disable-tunnel: [w393 w398] -> w384
          frame Disabled {
            n112 = Flush Queue(queue=w394, error in (no error)=w397) -> (queue out=w395:refnum<queue>, error out=w396:errorcluster)  [unwired: 1 out]
            n113 = Release Queue(queue=w395, error in (no error)=w396) -> (error out=w393:errorcluster)  [unwired: 1 in, 2 out]
          }
          frame Enabled {
          }
        }
      }
      frame "STOP" {
        n114 = disable-structure shown="Disabled" {
          disable-tunnel: w399 -> [w413 _]
          frame Disabled {
            n115 = Bundle("State"=Stack_Track."STOP", "Data 16"=u16[][] [], "Save to:"=path "C:/_DATA/test.tiff") -> (w415:T14)  [unwired: 1 in]
            n116 = Enqueue Element(queue=w413, element=w415) -> ()  [unwired: 2 in, 3 out]
          }
          frame Enabled {
          }
        }
        n117 = call <userlib>:"tm_stopcapture.vi"("error in (no error)"=w410) -> ("error out"=w409:errorcluster, "Handle out"=w412:u32)  [unwired: 9 in]
        n118 = call <userlib>:"tm_unpreparecapture.vi"("error in (no error)"=w409, "Handle in"=w412) -> ("error out"=w408:errorcluster, "Handle out"=w411:u32)  [unwired: 8 in]
        n119 = call <userlib>:"tm_closecamera.vi"("error in (no error)"=w408, "Handle in"=w411) -> ("error out"=w407:errorcluster)  [unwired: 9 in]
        n120 = call <userlib>:"tm_deinitialize.vi"("error in (no error)"=w407) -> ("error out"=w406:errorcluster)  [unwired: 10 in]
        n121 = disable-structure shown="Enabled" {
          disable-tunnel: w406 -> [w422 w423]
          disable-tunnel: w405 -> [w419 _]
          disable-tunnel: [w418 w423] -> w404
          frame Disabled {
            n122 = Flush Queue(queue=w419, error in (no error)=w422) -> (queue out=w420:refnum<queue>, error out=w421:errorcluster)  [unwired: 1 out]
            n123 = Release Queue(queue=w420, error in (no error)=w421) -> (error out=w418:errorcluster)  [unwired: 1 in, 2 out]
          }
          frame Enabled {
          }
        }
      }
      frame "Trigger Source" {
        (unwired) u32 1066144 items=["SENSOR MODE"=4212128, "CCD MODE"=4212384, "READOUT MODE"=4211872, "ACTIVE VIEW INDEX"=4343136, "BITS PER CHANNEL"=4342976, "IMAGE PIXEL TYPE"=4343296, "BINNING"=4215968, "EXPOSURE TIME"=2049184, "CONTRAST GAIN"=3163312, "CONTRAST OFFSET"=3163328, "LIGHT MODE"=2114720, "SENSITIVITY"=2114992, "PHOTON IMAGING MODE"=2115200, "HIGH DYNAMIC RANGE MODE"=3163360, "WHITE BALANCE"=3163568, "TEMPERATURE"=2115232, "TEMPERATURE TARGET"=2115264, "SENSOR COOLER FAN"=2115296, "LINEBUNDLE HEIGHT"=4212192, "MECHANICAL SHUTTER"=2115488, "BACK FOCUS POSITION"=8422304, "TRIGGER CONNECTOR"=1066432, "TRIGGER SOURCE"=1066144, "OUTPUT TRIGGER SOURCE"=1852576, "TRIGGER GLOBAL EXPOSURE"=2049680, "FIRST TRIGGER BEHAVIOR"=2049696, "CHANNEL SYNC"=1852352, "READOUT DIRECTION"=4211904, "PRE HSYNC COUNT"=1852704, "INTERNAL LINE SPEED"=4226000, "INTERNAL LINE INTERVAL"=4226016] ("Parameter")
        w432 = 1 items=["Snap", "Sequence"] ("Capture mode")
        n124 = Unbundle By Name(w426) -> ("Mode"=w425:T15)
        n125 = case shown="\"Brightfield\"" w425 {
          tunnel: [T12 {"Mode"=2, "Polarity"=2, "Times"=2, "Delay"=0.0} ("Parameters") T12 {"Mode"=2, "Polarity"=2, "Times"=2, "Delay"=0.0} ("Parameters") T12 {"Mode"=2, "Polarity"=2, "Times"=2, "Delay"=0.0} ("Parameters") T12 {"Mode"=1, "Polarity"=2, "Times"=2, "Delay"=0.0} ("Parameters") T12 {"Mode"=1, "Polarity"=2, "Times"=2, "Delay"=0.0} ("Parameters") T12 {"Mode"=1, "Polarity"=2, "Times"=2, "Delay"=0.0} ("Parameters")] -> w429
          tunnel: [CameraControlTypeDef."Preview" ("Enum") CameraControlTypeDef."Preview" ("Enum") CameraControlTypeDef."Preview" ("Enum") CameraControlTypeDef."Preview" ("Enum") CameraControlTypeDef."Preview" ("Enum") CameraControlTypeDef."Preview" ("Enum")] -> w424
          frame "XY", Default {
          }
          frame "XYZT" {
          }
          frame "XYZ" {
          }
          frame "XYZC" {
          }
          frame "X" {
          }
          frame "Brightfield" {
          }
        }
        n126 = call <userlib>:"tm_stopcapture.vi"("error in (no error)"=w433, "Handle in"=w436) -> ("error out"=w440:errorcluster, "Handle out"=w441:u32)  [unwired: 8 in]
        n127 = call <userlib>:"tm_unpreparecapture.vi"("error in (no error)"=w440, "Handle in"=w441) -> ("error out"=w428:errorcluster, "Handle out"=w431:u32)  [unwired: 8 in]
        n128 = call <userlib>:"tm_setinputtrigger.vi"("error in (no error)"=w428, "Parameters"=w429, "Handle in"=w431) -> ("error out"=w427:errorcluster, "Handle out"=w430:u32)  [unwired: 7 in]
        n129 = call <userlib>:"tm_preparecapture.vi"("error in (no error)"=w427, "Capture mode"=w432, "Handle in"=w430) -> ("error out"=w439:errorcluster, "Buffer Info"=w437:T9, "Handle out"=w438:u32)  [unwired: 5 in, 1 out]
        n130 = call <userlib>:"tm_startcapture_b.vi"("error in (no error)"=w439, "Handle in"=w438) -> ("error out"=w434:errorcluster, "Handle out"=w435:u32)  [unwired: 8 in]
      }
    }
    n131 = call "FPS_Counter.vi"("Array in"=w33) -> ("Array out"=w32:u32[], "Numeric"=→"FPS":dbl)  [unwired: 1 in]
    n132 = Unbundle By Name(w44) -> ("status"=→"Failed":bool)
    n133 = case shown="False" w46 {
      tunnel: w40 -> [w456 _]
      tunnel: w38 -> [_ w458]
      tunnel: w39 -> [w455 _]
      tunnel: [w455 w457] -> w37
      tunnel: [w456 w458] -> w36
      tunnel: w35 -> [_ w457]
      frame False {
      }
      frame True {
      }
    }
  }
  "error IO" <- w17
  n134 = while "Tiff Consumer" {
    tunnel: w14 -> [w482]
    shift-right: [w468] -> _
    shift-left: w6 -> [w467]
    shift-right: [w479] -> _
    shift-left: u32[] [] ("Array out") -> [w480]
    shift-right: [w465] -> _
    shift-left: _ -> [w466]
    shift-right: [w478] -> _
    shift-left: T6 {"State"=enum."Display", "Image"=[[0]], "Path"=path ""} ("input cluster") -> [w477]
    shift-right: [w461] -> _
    shift-left: w11 -> [w464]
    stop <- w473 stop-if-true
    # "Delay, maybe?\nCheck"
    n135 = Dequeue Element(queue=w482, timeout in ms (-1)=1) -> (element=w478:T6)  [unwired: 1 in, 3 out]
    n136 = Unbundle By Name(w477) -> ("State"=w481:T7, "Image"=w475:u16[][], "Path"=w474:path)
    n137 = call "IMAQ Copy"("Image Dst"=w464, "Image Src"=w467) -> ("Image Dst Out"=w461:T1)  [unwired: 4 in, 1 out]
    n138 = case shown="True" "Auto Contrast" {
      tunnel: [w484 w494] -> w472
      tunnel: w461 -> [w492 _]
      frame True {
        n139 = call "IMAQ Histogram"("Image"=w492) -> ("Histogram Report"=w493:T16)  [unwired: 9 in, 1 out]
        n140 = Unbundle(w493) -> ("Starting Value"=→"Maximal Value":sgl, "Mean Value"=w489:sgl, "Standard  Variation"=w488:sgl)  [unwired: 5 out]
        n141 = Multiply(x=w488, y=sgl 3.0) -> (x*y=w490:sgl)
        n142 = Add(x=w489, y=w490) -> (x+y=w486:sgl)
        n143 = disable-structure shown="Enabled" {
          frame Disabled {
            n144 = property on="Histogram" class="WFGraph (strict)" props=["Cursor", "Cursor X"]() -> ()  [unwired: 3 in, 2 out]
          }
          frame Enabled {
          }
        }
        n145 = Multiply(x=w486, y=sgl 2.0) -> (x*y=w484:sgl)
      }
      frame False {
        n146 = property on="Histogram" class="WFGraph (strict)"() -> ("Cursor.Cursor X"=w494:dbl)  [unwired: 2 in, 2 out]
      }
    }
    n147 = case shown="\"Idle\", Default" w481 {
      tunnel: w475 -> [w497 _ _ w524]
      tunnel: w467 -> [w501 w509 w513 w523]
      tunnel: [w504 w506 errorcluster {"status"=FALSE, "code"=0, "source"=""} ("error out") w522] -> _
      tunnel: [w500 w509 w513 w520] -> w468
      tunnel: w480 -> [w503 w508 w512 w521]
      tunnel: [w502 w508 w512 w521] -> w479
      tunnel: w474 -> [_ _ _ _]
      tunnel: [_ TRUE _ _] -> w473
      tunnel: w466 -> [w499 w506 _ _]
      tunnel: "Image Folder" -> [w496 w505 w510 w515]
      tunnel: [w496 w505 w510 w514] -> w459
      frame "Display" {
        n148 = call "IMAQ ArrayToImage"("Image Pixels (U16)"=w497, "error in (no error)"=w499, "Image"=w501) -> ("error out"=w504:errorcluster, "Image Out"=w500:T1)  [unwired: 7 in]
        n149 = Wait (ms)(milliseconds to wait=u32 40) -> ()  [unwired: 1 out]
        n150 = call "FPS_Counter.vi"("Array in"=w503) -> ("Array out"=w502:u32[])  [unwired: 1 in, 1 out]
      }
      frame "STOP" {
      }
      frame "Idle", Default {
      }
      frame "Save Image" {
        n151 = call "IMAQ ArrayToImage"("Image Pixels (U16)"=w524, "Image"=w523) -> ("error out"=w522:errorcluster, "Image Out"=w520:T1)  [unwired: 8 in]
        n152 = flat-sequence {
          tunnel: w522 -> [w527]
          tunnel: w520 -> [w528]
          tunnel: [w529] -> w519
          tunnel: [w525] -> w518
          tunnel: [w528] -> w517
          tunnel: [w527] -> w516
          tunnel: w515 -> [w526]
          tunnel: [w525] -> w514
          tunnel: w519 -> [w536]
          tunnel: w518 -> [w535]
          tunnel: w517 -> [w534]
          tunnel: w516 -> [w533]
          frame #0 {
            n153 = call "Create File with Incrementing Suffix Fast.vi"("disable buffering (F)"=TRUE, "format string (\" (%d)\")"="_%05d" ("format string (\" (%d)\")"), "file path"=w526) -> ("actual path"=w525:path, "refnum out"=w529:refnum<file>)  [unwired: 6 in, 1 out]
          }
          frame #1 {
            n154 = call-poly "IMAQ Write File 2"("error in (no error)"=w533, "File Path"=w535, "Image"=w534) -> ("error out"=w532:errorcluster)  [unwired: 7 in, 1 out]
            n155 = Close File(refnum=w536, error in=w532) -> ()  [unwired: 2 out]
          }
          frame #2 {
          }
        }
      }
    }
    "Image Path" <- w459
    n156 = Divide(x=65536.0, y=w472) -> (x/y=w470:dbl)
    n157 = call "IMAQ Multiply"("Image Src A"=w461, "Constant"=w470) -> ("Image Dst Out"=w469:T1)  [unwired: 5 in, 1 out]
    n158 = call "IMAQ Histograph"("error in (no error)"=w466, "Image"=w467) -> ("error out"=w465:errorcluster, "Histogram Graph"=→"Histogram":T2)  [unwired: 6 in, 2 out]
    n159 = case shown="True" "Display?" {
      tunnel: w469 -> [_ w495]
      frame False {
      }
      frame True {
        "Image" <- w495
      }
    }
  }
  n160 = disable-structure shown="Enabled" {
    disable-tunnel: "Camera Queue" -> [w538 _]
    disable-tunnel: w1 -> [w537 _]
    frame Disabled {
      n161 = while {
        tunnel: w538 -> [w540]
        tunnel: w537 -> [w541]
        stop <- w539 stop-if-true
        n162 = event shown="[0] Timeout" {
          selector: _ -> [_ _]
          dyn-events: _ -> [_ _]
          timeout: _ -> [_ _]
          tunnel: w541 -> [_ w545]
          tunnel: w540 -> [_ w544]
          tunnel: [_ TRUE] -> w539
          event Timeout {
            n163 = event-data() -> ()  [unwired: 1 in, 3 out]
          }
          event Panel Close {
            n164 = event-data() -> ()  [unwired: 1 in, 4 out]
            n165 = Bundle("Enum"=CameraControlTypeDef."Close", "Microscope Settings"=w545) -> (w543:cluster{"Enum":T8, "Microscope Settings":T3})  [unwired: 1 in]
            n166 = Enqueue Element(queue=w544, element=w543) -> ()  [unwired: 2 in, 3 out]
          }
        }
      }
    }
    frame Enabled {
    }
  }
